vi "overwriteTDMSTest.vi"() -> ()   [LabVIEW 2018]
panel:
  out "data 2":cluster{"cmd":string, "val":i32[]}
  out "data":waveform(sgl)
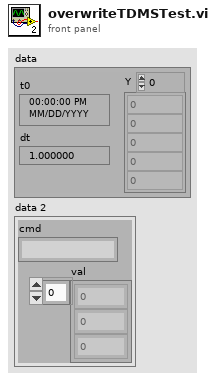
[diagram p1: front panel]
types:
  T1 = enum16{"open", "replace", "create", "open or create", "replace or create", "replace or create with confirmation"}
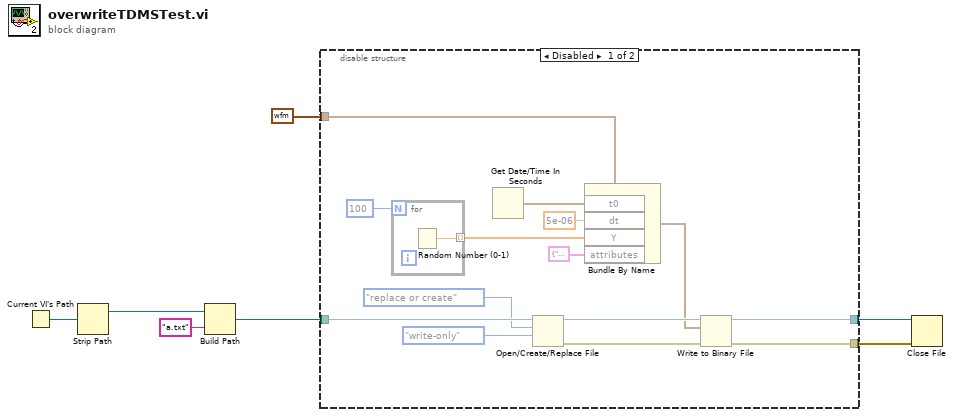
[diagram p0: block diagram]
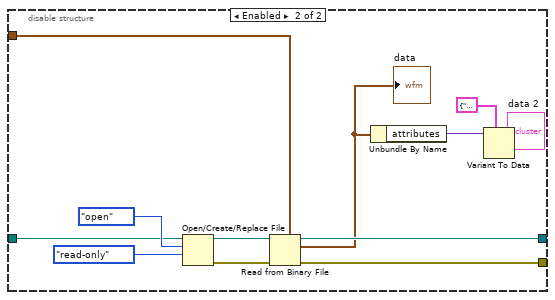
[diagram p2: hidden frame]
diagram:
  n1 = Current VI's Path() -> (path=w7:path)
  n2 = Strip Path(path=w7) -> (stripped path=w1:path)  [unwired: 1 out]
  n3 = Build Path(base path=w1, name or relative path="a.txt") -> (appended path=w2:path)
  n4 = disable-structure shown="Disabled" {
    disable-tunnel: w2 -> [w16 w32]
    disable-tunnel: waveform(sgl) {"t0"=timestamp(0 s since 1904-01-01), "dt"=1.0, "Y"=[]} ("SignalData") -> [w11 w27]
    disable-tunnel: [w9 w28] -> w4
    disable-tunnel: [w8 w29] -> w3
    frame Disabled {
      n5 = for {
        N: 100 -> [_]
        tunnel: [w22] -> w18 mode=indexing
        n6 = Random Number (0-1)() -> (number: 0 to 1=w22:dbl)
      }
      n7 = Get Date/Time In Seconds() -> (seconds since 1Jan1904=w21:timestamp)
      n8 = Open/Create/Replace File(file path (use dialog)=w16, operation (0:open)=T1."replace or create", access (0:read/write)=enum16{"read/write", "read-only", "write-only"}."write-only") -> (refnum out=w14:refnum<file>, error out=w13:errorcluster)  [unwired: 3 in, 1 out]
      n9 = Bundle By Name(cluster=w11, "t0"=w21, "dt"=5e-06, "Y"=w18, "attributes"=cluster{"cmd":string, "val":i32[]} {"cmd"="", "val"=[1, 2, 3]} ("attr")) -> (w12:waveform(sgl))
      n10 = Write to Binary File(file (use dialog)=w14, data=w12, error in=w13) -> (refnum out=w9:refnum<file>, error out=w8:errorcluster)  [unwired: 3 in, 1 out]
    }
    frame Enabled {
      n11 = Open/Create/Replace File(file path (use dialog)=w32, operation (0:open)=T1."open", access (0:read/write)=enum16{"read/write", "read-only", "write-only"}."read-only") -> (refnum out=w31:refnum<file>, error out=w30:errorcluster)  [unwired: 3 in, 1 out]
      n12 = Read from Binary File(5:w27, 8:w30, 11:w31) -> (0:w29:errorcluster, 2:w26:waveform(sgl), 3:w28:refnum<file>)  [unwired: 3 in, 1 out]
      "data" <- w26
      n13 = Unbundle By Name(w26) -> ("attributes"=w25:variant)
      n14 = Variant To Data(type=cluster{"cmd":string, "val":i32[]} {"cmd"="", "val"=[1, 2, 3]} ("attr"), Variant=w25) -> (data=→"data 2":cluster{"cmd":string, "val":i32[]})  [unwired: 1 in, 1 out]
    }
  }
  n15 = Close File(refnum=w4, error in=w3) -> ()  [unwired: 2 out]
